vi "lsl time correction ex.vi"(0 "in":cluster{}, 1 "ec":i32, 5 "remote_time":dbl, 7 "uncertainty":dbl, 9 "timeout":dbl, 11 "error in (no error)":errorcluster) -> (3 "ec out":i32, 4 "in out":cluster{}, 6 "remote_time out":dbl, 8 "uncertainty out":dbl, 10 "function return":dbl, 15 "error out":errorcluster)   [LabVIEW 2018, in "liblsl-LabVIEW.lvlib"]
doc: "extern LIBLSL_C_API double lsl_time_correction_ex(lsl_inlet in, double *remote_time, double *uncertainty, double timeout, int32_t *ec);"
uses:
  <userlib>/liblsl-LabVIEW/liblsl-LabVIEW.lvlib
  <userlib>/liblsl-LabVIEW/liblsl64.dll
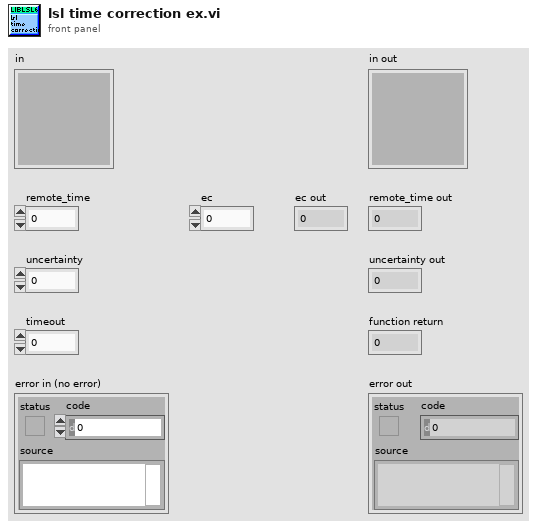
[diagram p1: front panel]
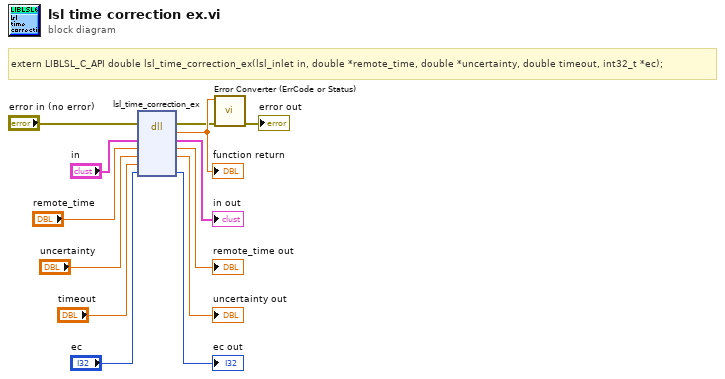
[diagram p0: block diagram]
diagram:
  # "extern LIBLSL_C_API double lsl_time_correction_ex(lsl_inlet in, double *remote_time, double *uncertainty, double timeout, int32_t *ec);"
  n1 = dll-call lib="C:/Program Files/National Instruments/LabVIEW 2018/user.lib/liblsl-LabVIEW/liblsl64.*" fn="lsl_time_correction_ex"(error in="error in (no error)", "in"="in", "remote_time"="remote_time", "uncertainty"="uncertainty", "timeout"="timeout", "ec"="ec") -> (error out=w2:errorcluster, w13:dbl, "in"=→"in out":cluster{}, "remote_time"=→"remote_time out":dbl, "uncertainty"=→"uncertainty out":dbl, "ec"=→"ec out":i32)  [unwired: 3 in, 1 out]
  "function return" <- w13
  n2 = call <userlib>:"Error Converter (ErrCode or Status).vi"("error in (no error)"=w2, "error code"=w13) -> ("error out"=→"error out":errorcluster)  [unwired: 9 in]
